vi "INTELLIFAUCET AO Control.vi"(0 "VISA session":refnum<visa-resource-name>="MW100", 5 "HEWH MW100 Channel Numbers":T1="001", 7 "Output Value (0)":i32, 11 "Error In":errorcluster, 12 "Debug":bool, 13 "milliseconds to wait":u32=100) -> (4 "dup VISA session":refnum<visa-resource-name>, 15 "error out":errorcluster)   [LabVIEW 2023]
uses:
  MW100/Type Definitions/HEWH MW100 Channel Numbers.ctl
panel:
  in  "Retries Allowed":i32=3
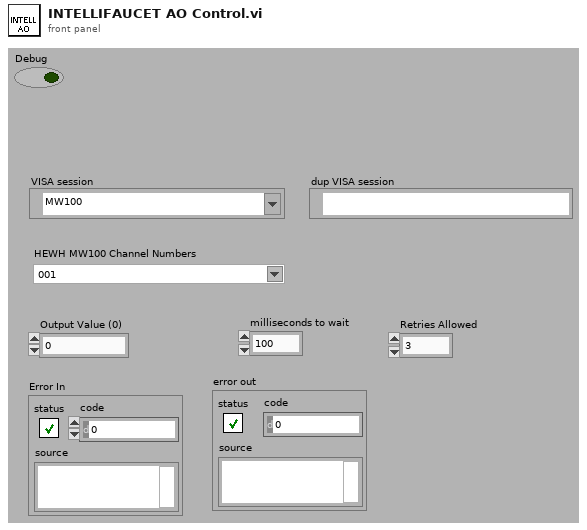
[diagram p1: front panel]
types:
  T1 = typedef "HEWH MW100 Channel Numbers.ctl" = string
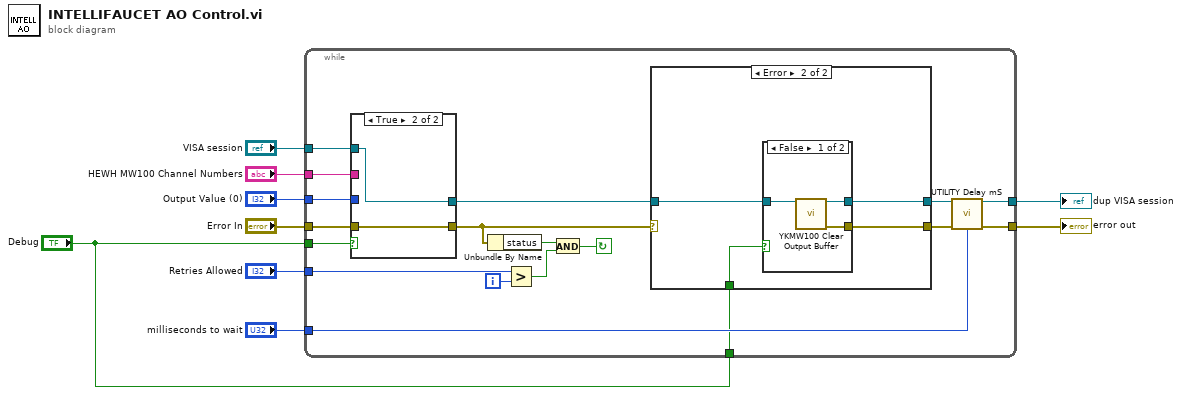
[diagram p0: block diagram]
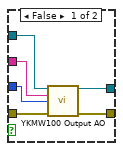
[diagram p2: hidden frame]
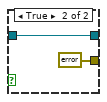
[diagram p4: hidden frame]
diagram:
  n1 = while {
    tunnel: "HEWH MW100 Channel Numbers" -> [w26]
    tunnel: "Output Value (0)" -> [w25]
    tunnel: "Error In" -> [w20]
    tunnel: [w13] -> w6
    tunnel: [w21] -> w9
    tunnel: "VISA session" -> [w24]
    tunnel: "Retries Allowed" -> [w16]
    tunnel: "milliseconds to wait" -> [w12]
    tunnel: "Debug" -> [w11]
    tunnel: "Debug" -> [w10]
    i -> [w18]
    stop <- w23 continue-if-true
    n2 = case shown="True" w11 {
      tunnel: w26 -> [w32 _]
      tunnel: w25 -> [w31 _]
      tunnel: w24 -> [w30 w34]
      tunnel: w20 -> [w29 w33]
      tunnel: [w28 w33] -> w19
      tunnel: [w27 w34] -> w14
      frame False {
        n3 = call "YKMW100 Output AO.vi"("VISA session"=w30, "Channel String (001)"=w32, "Output Value (0)"=w31, "error in (no error)"=w29) -> ("dup VISA session"=w27:refnum<visa-resource-name>, "error out"=w28:errorcluster)  [unwired: 10 in]
      }
      frame True {
      }
    }
    n4 = Unbundle By Name(w19) -> ("status"=w22:bool)
    n5 = Greater?(x=w16, y=w18) -> (0:w17:bool)
    n6 = And(x=w22, y=w17) -> (x .and. y?=w23:bool)
    n7 = case shown="Error" w19 {
      selector: w19 -> [w36 _]
      tunnel: w14 -> [w35 w40]
      tunnel: [w36 w38] -> w15
      tunnel: [w35 w39] -> w13
      tunnel: w10 -> [_ w37]
      frame No Error {
      }
      frame Error {
        n8 = case shown="False" w37 {
          tunnel: w40 -> [w43 w45]
          tunnel: [w42 w45] -> w39
          tunnel: [w41 errorcluster {"status"=FALSE, "code"=0, "source"=""} ("error out")] -> w38
          frame False {
            n9 = call "YKMW100 Clear Output Buffer.vi"("VISA session"=w43) -> ("dup VISA session"=w42:refnum<visa-resource-name>, "error out"=w41:errorcluster)  [unwired: 13 in]
          }
          frame True {
          }
        }
      }
    }
    n10 = call "UTILITY Delay mS.vi"("Error In"=w15, "milliseconds to wait"=w12) -> ("Error Out"=w21:errorcluster)  [unwired: 13 in]
  }
  "error out" <- w9
  "dup VISA session" <- w6
